vi "Error UI (Kyle Green's conflicted copy 2012-06-09).vi"() -> ()   [LabVIEW 2011]
uses:
  <vilib>/Platform/TimedLoop/XDataNode/XDataNode.xnode
  <vilib>/Platform/TimedLoop/XDataNode/nitl_modes.ctl
  <vilib>/Platform/TimedLoop/XDataNode/XDNodeRunTimeDep.lvlib
  <vilib>/Platform/TimedLoop/XDataNode/wakeup.ctl
  <vilib>/Platform/TimedLoop/XDataNode/timing_clust.ctl
  <vilib>/Instr/_visa.llb/VISA Configure Serial Port (Instr).vi
panel:
  out "Error":bool
  out "OK":bool
  in  "stop?":bool
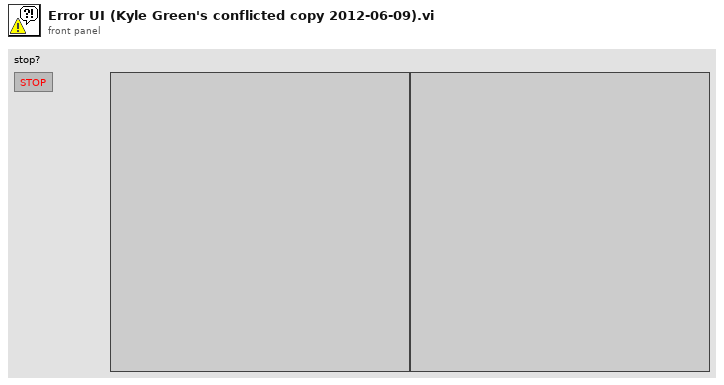
[diagram p1: front panel]
types:
  T1 = typedef "XDNodeRunTimeDep.lvlib/timing_clust.ctl" = cluster{"Expected End [f-1]":u64, "Actual End [f-1]":u64, "Finished Late? [f-1]":bool, "Expected End [i-1]":u64, "Actual End [i-1]":u64, "Finished Late? [i-1]":bool, "Expected Start [i]":u64, "Actual Start [i]":u64, "Expected Start [f]":u64, "Actual Start [f]":u64, "Source Name":string, "Structure Name":string, "Period":i64, "Deadline":i64, "Offset":i64, "Start":i64, "Priority":i32, "Timeout":i32, "Mode":T2, "Wakeup Reason":T3, "Error":errorcluster, "Source Type":string, "Secondary Source Type":string, "Global End Time":u64, "Global Start Time":u64, "Frame Duration":u64, "Iteration Duration":u64, "Assigned CPU":i32, "I/O Scan Engine Mode":u32}
  T2 = typedef "XDNodeRunTimeDep.lvlib/nitl_modes.ctl" = enum32{"No Change", "Process missed periods, maintain original phase", "Discard missed periods, maintain original phase", "Process missed periods, ignore original phase", "Discard missed periods, ignore original phase"}
  T3 = typedef "XDNodeRunTimeDep.lvlib/wakeup.ctl" = enum32{"Normal", "Aborted", "Asynchronous wakeup", "Timing source error", "Timed loop error", "Timeout"}
  T4 = enum16{"Idle", "Wiimote", "Joypad", "IGVC", "Avoide Objects", "Avoide Lines", "Path Planning", "Heading", "Waypoint"}
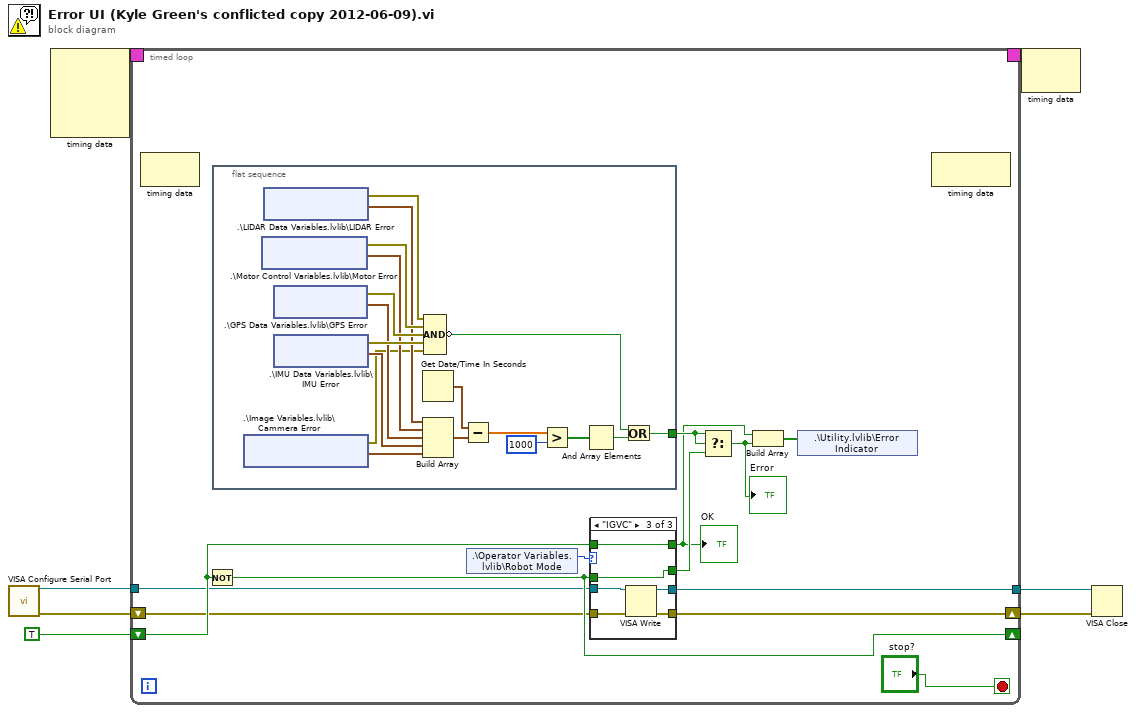
[diagram p0: block diagram]
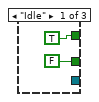
[diagram p2: hidden frame]
diagram:
  n1 = call-poly "VISA Configure Serial Port"() -> ("VISA resource name out"=w3:refnum<visa-resource-name>, "error out"=w4:errorcluster)  [unwired: 14 in]
  n2 = node-c288() -> (w7:T1)  [unwired: 4 in]
  n3 = timed-loop {
    timing: w7 -> [_]
    timing-out: [_] -> w6
    shift-right: [w14] -> _
    shift-left: TRUE ("logical AND") -> [w16]
    shift-right: [w11] -> w1
    shift-left: w4 -> [w10]
    tunnel: w3 -> [w9]
    tunnel: [w8] -> w2
    stop <- "stop?" stop-if-true
    n4 = node-c288() -> ()  [unwired: 1 in, 1 out]
    n5 = Not(x=w16) -> (.not. x?=w14:bool)
    n6 = flat-sequence {
      tunnel: [w33] -> w19
      frame #0 {
        n7 = shared-variable ".\\Image Variables.lvlib\\Cammera Error"() -> (w32:errorcluster, w31:timestamp)  [unwired: 1 in, 1 out]
        n8 = shared-variable ".\\Motor Control Variables.lvlib\\Motor Error"() -> (w47:errorcluster, w42:timestamp)  [unwired: 1 in, 1 out]
        n9 = shared-variable ".\\LIDAR Data Variables.lvlib\\LIDAR Error"() -> (w48:errorcluster, w43:timestamp)  [unwired: 1 in, 1 out]
        n10 = shared-variable ".\\GPS Data Variables.lvlib\\GPS Error"() -> (w46:errorcluster, w41:timestamp)  [unwired: 1 in, 1 out]
        n11 = shared-variable ".\\IMU Data Variables.lvlib\\IMU Error"() -> (w45:errorcluster, w40:timestamp)  [unwired: 1 in, 1 out]
        n12 = Get Date/Time In Seconds() -> (seconds since 1Jan1904=w39:timestamp)
        n13 = Build Array(w43, w42, w41, w40, w31) -> (w38:timestamp[])
        n14 = Compound Arithmetic op=AND(w48, w47, w46, w45, w32) -> (invert w44:bool)
        n15 = Subtract(x=w39, y=w38) -> (x-y=w37:dbl[])
        n16 = Greater?(x=w37, y=1000) -> (0:w35:bool[])
        n17 = And Array Elements(Boolean array=w35) -> (logical AND=w34:bool)
        n18 = Or(x=w44, y=w34) -> (x .or. y?=w33:bool)
      }
    }
    n19 = shared-variable ".\\Operator Variables.lvlib\\Robot Mode"() -> (w17:T4)  [unwired: 1 in, 1 out]
    n20 = case shown="\"IGVC\"" w17 {
      tunnel: [TRUE ("logical AND") w24 w30] -> w13
      tunnel: w16 -> [_ w24 w30]
      tunnel: [FALSE w23 w29] -> w15
      tunnel: w14 -> [_ w23 w29]
      tunnel: [_ _ w28] -> w11
      tunnel: w10 -> [_ _ w27]
      tunnel: w9 -> [_ _ w26]
      tunnel: [_ _ w25] -> w8
      frame "Idle" {
      }
      frame "Wiimote", Default {
      }
      frame "IGVC" {
        n21 = VISA Write(VISA resource name=w26, error in (no error)=w27) -> (VISA resource name out=w25:refnum<visa-resource-name>, error out=w28:errorcluster)  [unwired: 1 in, 1 out]
      }
    }
    "OK" <- w13
    n22 = Select(t=w19, s=w19, f=w15) -> (s? t:f=w12:bool)
    "Error" <- w12
    n23 = Build Array(w13, w12) -> (w18:bool[])
    n24 = shared-variable ".\\Utility.lvlib\\Error Indicator"(w18) -> ()  [unwired: 1 in, 1 out]
    n25 = node-c288() -> ()  [unwired: 1 in, 1 out]
  }
  n26 = node-c288(w6) -> ()  [unwired: 1 out]
  n27 = VISA Close(VISA resource name=w2, error in (no error)=w1) -> ()  [unwired: 1 out]
